vi "AOTF_Digital_Pulse_Switch.vi"(7 "Number of active lines":u8, 8 "AOTF-Digital out":tag="Dev2/port0", 9 "AOTF-Digital switch in":tag="/Dev1/PFI1", 10 "Pictures per pixel":u8, 11 "Pulse per Wavelength":u8[](array[numeric])) -> (0 "error out":errorcluster, 3 "task out":refnum<k21>)   [LabVIEW 2011]
uses:
  <vilib>/DAQmx/write.llb/DAQmx Write (Digital 1D U8 1Chan NSamp).vi
  <vilib>/DAQmx/create/channels.llb/DAQmx Create Channel (DO-Digital Output).vi
  <vilib>/DAQmx/configure/timing.llb/DAQmx Timing (Sample Clock).vi
  <vilib>/DAQmx/miscellaneous.llb/DAQmx Fill In Error Info.vi
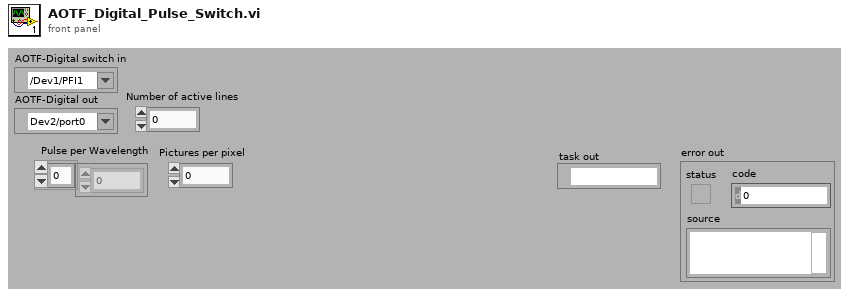
[diagram p1: front panel]
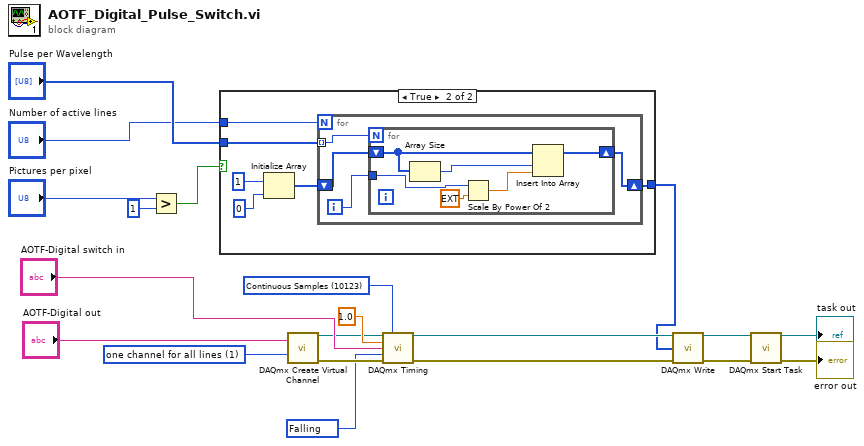
[diagram p0: block diagram]
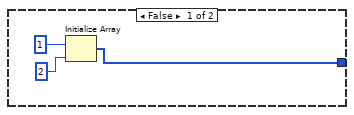
[diagram p2: hidden frame]
diagram:
  w7 = 10171 items=["Rising"=10280, "Falling"=10171] ("active edge")
  w6 = 10123 items=["Finite Samples"=10178, "Continuous Samples"=10123, "Hardware Timed Single Point"=12522] ("sample mode")
  w10 = 1 items=["one channel for each line", "one channel for all lines"] ("line grouping")
  n1 = Greater?(x="Pictures per pixel", y=u8 1) -> (0:w2:bool)
  n2 = case shown="True" w2 {
    tunnel: "Number of active lines" -> [_ w29]
    tunnel: "Pulse per Wavelength" -> [_ w28]
    tunnel: [w21 w24] -> w5
    frame False {
      n3 = Initialize Array(1 ("element"), 2 ("dimension size")) -> (w21:i32[])
    }
    frame True {
      n4 = Initialize Array(1 ("element"), 0 ("dimension size")) -> (w27:i32[])
      n5 = for {
        N: w29 -> [_]
        tunnel: w28 -> [w33] mode=indexing
        shift-right: [w31] -> w24
        shift-left: w27 -> [w32]
        i -> [w30]
        n6 = for {
          N: w33 -> [_]
          shift-right: [w39] -> w31
          shift-left: w32 -> [w38]
          tunnel: w30 -> [w35]
          n7 = Array Size(array=w38) -> (size(s)=w37:i32)
          n8 = Scale By Power Of 2(n=w35, x=ext 1.0) -> (x*2^n=w36:ext)
          n9 = Insert Into Array(array=w38, index=w37, new element=w36) -> (w39:i32[])
        }
      }
    }
  }
  n10 = call-poly <vilib>:"DAQmx Create Virtual Channel.vi"("lines"="AOTF-Digital out", "line grouping"=w10) -> ("task out"=w11:refnum<k21>, "error out"=w12:errorcluster)  [unwired: 5 in, 7 out]
  n11 = call-poly <vilib>:"DAQmx Timing.vi"("task/channels in"=w11, "sample mode"=w6, "rate"=1.0, "source"="AOTF-Digital switch in", "active edge"=w7, "error in"=w12) -> ("task out"=w9:refnum<k21>, "error out"=w8:errorcluster)  [unwired: 1 in, 7 out]
  n12 = call-poly <vilib>:"DAQmx Write.vi"("task/channels in"=w9, "data"=w5, "error in"=w8) -> ("task out"=w13:refnum<k21>, "error out"=w14:errorcluster)  [unwired: 1 in, 10 out]
  n13 = call <vilib>:"DAQmx Start Task.vi"("task/channels in"=w13, "error in"=w14) -> ("task out"=→"task out":refnum<k21>, "error out"=→"error out":errorcluster)  [unwired: 12 out]
